vi "Create SG Power Meter Accessor.vi"(0 "SG Path":refnum<class "SG Abstract Path.lvclass">, 11 "error in":errorcluster) -> (4 "SG Path PM Accessor out":refnum<class "SG Path PM Accessor Base.lvclass">, 15 "error out":errorcluster)   [LabVIEW 2023, in "RFFixtureCharact.Instruments.lvlib" / "Power Meter Factory.lvclass"]
uses:
  Power Meter Factory.lvclass
  SG Path PM Accessor Base/SG Path PM Accessor Base.lvclass
  Public/Base Classes/Scalar/SG Abstract Path/SG Abstract Path.lvclass
  SG Path Simulated PM Accessor/SG Path Simulated PM Accessor.lvclass
  C:/srd-semi-rfcal-software/AuxTools/STSRFFixtureCharactUtility/Source/Code Modules/Fixture/Instruments/Power Meter/SG Path PM Accessor Base/SG Path PM Accessor Base.lvclass
  Simulated/Simulated Power Meter.lvclass
  C:/srd-semi-rfcal-software/AuxTools/STSRFFixtureCharactUtility/Source/Code Modules/Fixture/Instruments/Power Meter/Power Meter Base/Power Meter Base.lvclass
  13e43a11-3f49-451d-9662-7e96f715d9cd.vi
  <vilib>/Utility/error.llb/Trim Whitespace One-Sided.vi
  Common/Data Cache/Settings Dictionary/Setting Keys.vi
  <vilib>/Comparison/Equal/Equal Functor/Equal Functor.lvclass
  Power Meter Base/Power Meter Base.lvclass
  Power Meter Factory.lvclass/Power Meter Factory.ctl
  Common/RFCalAndFixtureCharact.Common.lvlib
  C:/srd-semi-rfcal-software/AuxTools/STSRFFixtureCharactUtility/Source/Code Modules/Fixture/Instruments/Power Meter/SG Path Simulated PM Accessor/SG Path Simulated PM Accessor.lvclass
  C:/srd-semi-rfcal-software/AuxTools/STSRFFixtureCharactUtility/Source/Code Modules/Fixture/Instruments/Power Meter/Simulated/Simulated Power Meter.lvclass
  C:/srd-semi-rfcal-software/AuxTools/STSRFFixtureCharactUtility/Source/Code Modules/Fixture/Public/Base Classes/Scalar/Scalar Path/Scalar Path.lvclass
  C:/srd-semi-rfcal-software/AuxTools/STSRFFixtureCharactUtility/Source/Code Modules/Common/Base Classes/Path/Path.lvclass
  C:/srd-semi-rfcal-software/AuxTools/STSRFFixtureCharactUtility/Source/Code Modules/Fixture/Public/Base Classes/Scalar/SG Abstract Path/SG Abstract Path.lvclass
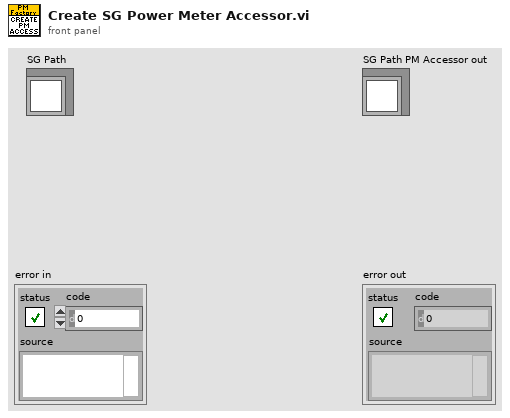
[diagram p1: front panel]
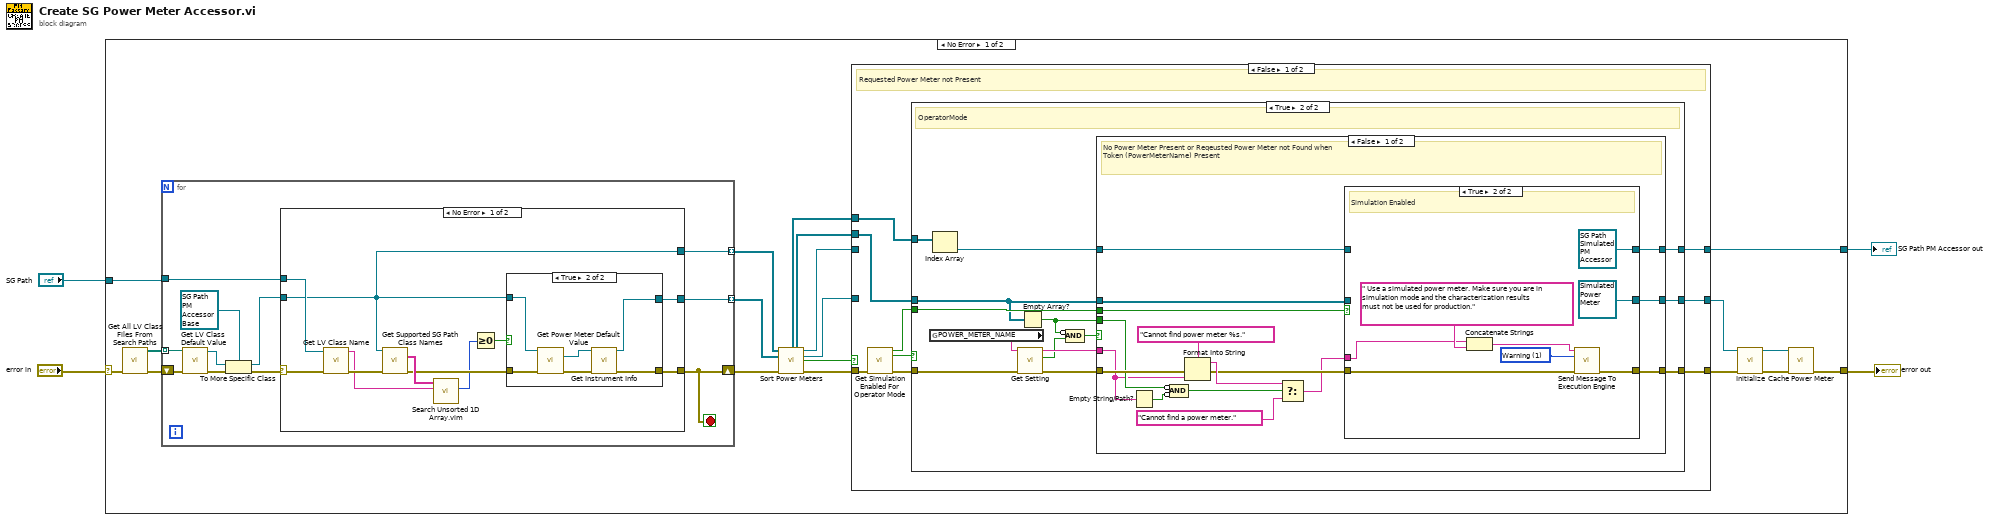
[diagram p0: block diagram]
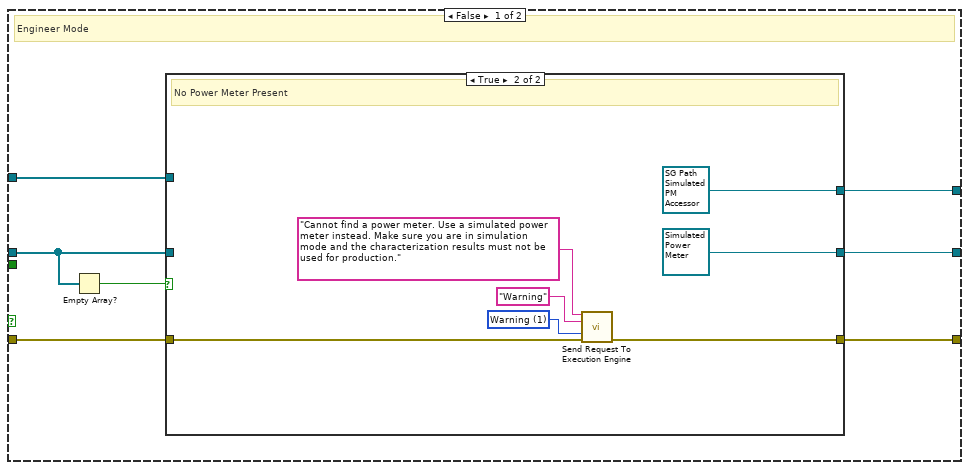
[diagram p2: hidden frame]
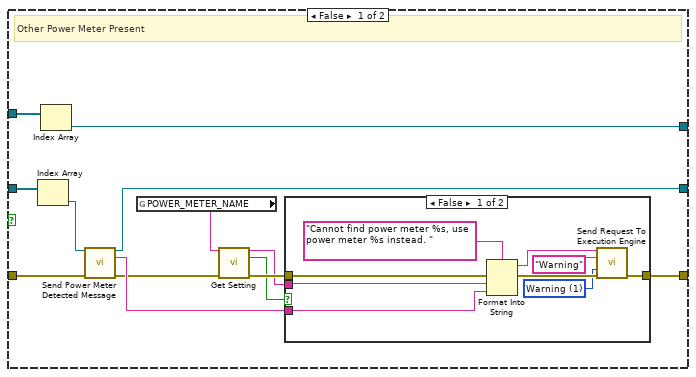
[diagram p3: hidden frame]
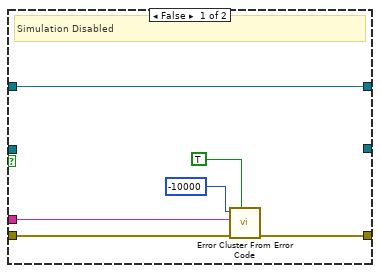
[diagram p5: hidden frame]
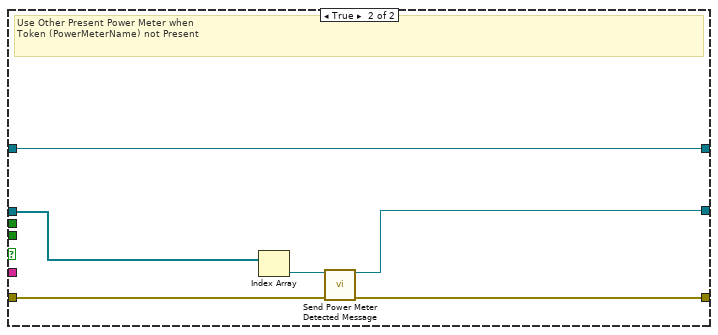
[diagram p6: hidden frame]
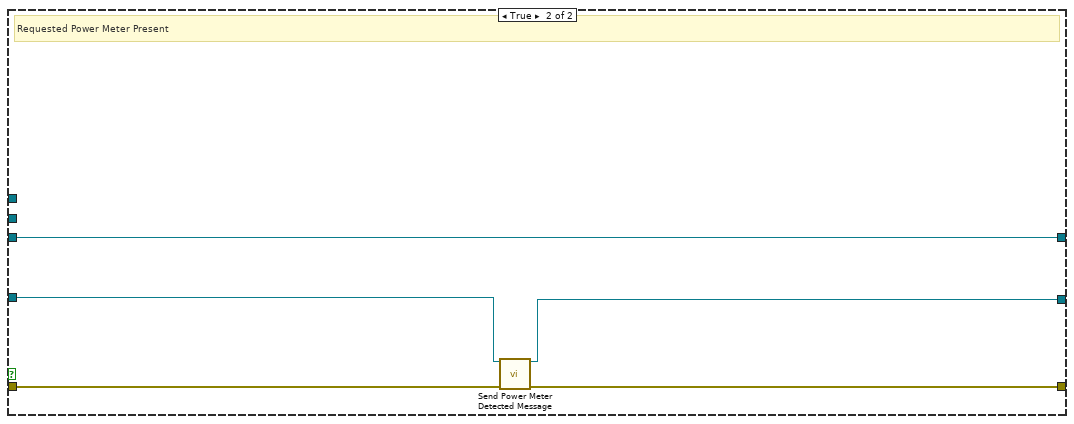
[diagram p7: hidden frame]
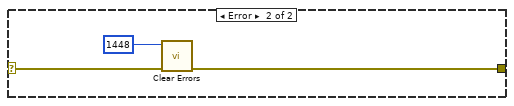
[diagram p9: hidden frame]
diagram:
  n1 = case shown="No Error" "error in" {
    selector: "error in" -> [w23 w157]
    tunnel: [w5 w157] -> w3
    tunnel: "SG Path" -> [w20 _]
    tunnel: [w19 _] -> w1
    frame No Error {
      n2 = call "Get All LV Class Files From Search Paths.vi"("error in (no error)"=w23) -> ("All Files in Dir"=w21:path[], "error out"=w22:errorcluster)  [unwired: 13 in]
      n3 = for {
        shift-right: [w128] -> w14
        shift-left: w22 -> [w135]
        tunnel: w21 -> [w133] mode=indexing
        tunnel: [w126] -> w17 mode=indexing
        tunnel: w20 -> [w129]
        tunnel: [w125] -> w18 mode=indexing
        stop <- w128 stop-if-true
        n4 = call <vilib>:"Get LV Class Default Value.vi"("error in (no error)"=w135, "class path"=w133) -> ("error out"=w134:errorcluster, "object"=w132:refnum<class>)  [unwired: 8 in]
        n5 = To More Specific Class(target class=refnum<class "SG Path PM Accessor Base.lvclass"> refnum ("RFFixtureCharact.Instruments.lvlib:SG Path PM Accessor Base.lvclass"), reference=w132, error in=w134) -> (specific class reference=w131:refnum<class "SG Path PM Accessor Base.lvclass">, error out=w130:errorcluster)
        n6 = case shown="No Error" w130 {
          selector: w130 -> [w146 w155]
          tunnel: [w142 w154] -> w128
          tunnel: w131 -> [w136 _]
          tunnel: [w143 _] -> w126
          tunnel: w129 -> [w145 _]
          tunnel: [w136 _] -> w125
          frame No Error {
            n7 = call <vilib>:"Get LV Class Name.vi"("error in (no error)"=w146, "object"=w145) -> ("error out"=w144:errorcluster, "class name"=w140:string)  [unwired: 8 in]
            n8 = call-dynamic "Get Supported SG Path Class Names.vi"("SG Path PM Accessor in"=w136, "error in"=w144) -> ("Supported SG Path Class Names"=w141:string[], "error out"=w139:errorcluster)  [unwired: 11 in, 1 out]
            n9 = call "Search Unsorted 1D Array.vim"("element"=w140, "unsorted 1D array"=w141) -> ("index of element"=w138:i32)  [unwired: 9 in]
            n10 = Greater Or Equal To 0?(x=w138) -> (x >= 0?=w137:bool)
            n11 = case shown="True" w137 {
              tunnel: w136 -> [_ w153]
              tunnel: [_ w151] -> w143
              tunnel: w139 -> [w147 w150]
              tunnel: [w147 w148] -> w142
              frame False {
              }
              frame True {
                n12 = call-dynamic "Get Power Meter Default Value.vi"("SG Path PM Accessor in"=w153, "error in (no error)"=w150) -> ("Power Meter out"=w149:refnum<class "Power Meter Base.lvclass">, "error out"=w152:errorcluster)  [unwired: 11 in, 1 out]
                n13 = call-dynamic "Get Instrument Info.vi"("Power Meter Base in"=w149, "error in (no error)"=w152) -> ("Power Meter Base out"=w151:refnum<class "Power Meter Base.lvclass">, "error out"=w148:errorcluster)  [unwired: 12 in]
              }
            }
          }
          frame Error {
            n14 = call <vilib>:"Clear Errors.vi"("error in (no error)"=w155, "specific error code to clear (0: all)"=1448) -> ("error out"=w154:errorcluster)  [unwired: 4 in, 1 out]
          }
        }
      }
      n15 = call "Sort Power Meters.vi"("SG Path PM Accessor Base Array in"=w18, "Power Meter Base Array in"=w17, "error in"=w14) -> ("All Present SG Path PMs Except Requested"=w13:refnum<class "SG Path PM Accessor Base.lvclass">[], "All Present PMs Except Requested"=w12:refnum<class "Power Meter Base.lvclass">[], "Requested SG Path PM Accessor"=w16:refnum<class "SG Path PM Accessor Base.lvclass">, "Requested PM"=w15:refnum<class "Power Meter Base.lvclass">, "Requested PM Found?"=w10:bool, "error out"=w11:errorcluster)  [unwired: 7 in]
      n16 = case shown="False" w10 {
        tunnel: [w32 w124] -> w19
        tunnel: [w31 w122] -> w7
        tunnel: w16 -> [_ w124]
        tunnel: w11 -> [w30 w123]
        tunnel: w15 -> [_ w121]
        tunnel: w13 -> [w25 _]
        tunnel: w12 -> [w26 _]
        tunnel: [w24 w120] -> w9
        frame False {
          # "Requested Power Meter not Present"
          n17 = call "Get Simulation Enabled For Operator Mode.vi"("error in (no error)"=w30) -> ("Use Simulated Instrument?"=w29:bool, "Use Operator Mode?"=w28:bool, "error out"=w27:errorcluster)  [unwired: 12 in]
          n18 = case shown="True" w28 {
            tunnel: w29 -> [_ w83]
            tunnel: w27 -> [w39 w76]
            tunnel: [w38 w82] -> w32
            tunnel: [w34 w81] -> w31
            tunnel: w26 -> [w36 w74]
            tunnel: w25 -> [w35 w80]
            tunnel: [w33 w78] -> w24
            frame False {
              # "Engineer Mode"
              n19 = Empty Array?(array=w36) -> (empty?=w37:bool)
              n20 = case shown="True" w37 {
                tunnel: w39 -> [w45 w66]
                tunnel: [w40 w69] -> w34
                tunnel: [w51 refnum<class "SG Path Simulated PM Accessor.lvclass"> refnum ("RFFixtureCharact.Instruments.lvlib:SG Path Simulated PM Accessor.lvclass")] -> w38
                tunnel: w36 -> [w44 _]
                tunnel: w35 -> [w52 _]
                tunnel: [w50 refnum<class "Simulated Power Meter.lvclass"> refnum ("PM Simulated in")] -> w33
                frame False {
                  # "Other Power Meter Present"
                  n21 = Index Array(array=w44) -> (element=w43:refnum<class "Power Meter Base.lvclass">)  [unwired: 1 in]
                  n22 = Index Array(array=w52) -> (element=w51:refnum<class "SG Path PM Accessor Base.lvclass">)  [unwired: 1 in]
                  n23 = call "Send Power Meter Detected Message.vi"("Power Meter in"=w43, "error in"=w45) -> ("Power Meter out"=w50:refnum<class "Power Meter Base.lvclass">, "Active Instrument Info String"=w42:string, "error out"=w41:errorcluster)  [unwired: 11 in]
                  n24 = global read "Setting Keys.vi" "POWER_METER_NAME"() -> (w49:string)
                  n25 = call "Get Setting.vi"("Setting name"=w49, "error in (no error)"=w41) -> ("Setting value out"=w46:string, "Setting empty or not found?"=w47:bool, "error out"=w48:errorcluster)  [unwired: 11 in]
                  n26 = case shown="False" w47 {
                    tunnel: w48 -> [w60 w62]
                    tunnel: w42 -> [w53 _]
                    tunnel: [w55 w62] -> w40
                    tunnel: w46 -> [w54 _]
                    frame False {
                      w56 = 1 items=["Info", "Warning", "Error", "Action"] ("Request Content Type")
                      n27 = Format Into String(format string="Cannot find power meter %s, use power meter %s instead. " ("message"), error in=w60, w54, w53) -> (resulting string=w58:string, error out=w57:errorcluster)  [unwired: 1 in]
                      n28 = call "Send Request To Execution Engine.vi"("Request Message"=w58, "Request Header"="Warning", "Request Content Type"=w56, "error in (no error)"=w57) -> ("error out"=w55:errorcluster)  [unwired: 10 in, 1 out]
                    }
                    frame True {
                    }
                  }
                }
                frame True {
                  w67 = 1 items=["Info", "Warning", "Error", "Action"] ("RequestContentType")
                  # "No Power Meter Present"
                  n29 = call "Send Request To Execution Engine.vi"("Request Message"="Cannot find a power meter. Use a simulated power meter instead. Make sure you are in simulation mode and the characterization results must not be used for production." ("message"), "Request Header"="Warning" ("headerText"), "Request Content Type"=w67, "error in (no error)"=w66) -> ("error out"=w69:errorcluster)  [unwired: 10 in, 1 out]
                }
              }
            }
            frame True {
              # "OperatorMode"
              n30 = global read "Setting Keys.vi" "POWER_METER_NAME"() -> (w77:string)
              n31 = Index Array(array=w80) -> (element=w79:refnum<class "SG Path PM Accessor Base.lvclass">)  [unwired: 1 in]
              n32 = call "Get Setting.vi"("Setting name"=w77, "error in (no error)"=w76) -> ("Setting value out"=w72:string, "Setting empty or not found?"=w71:bool, "error out"=w75:errorcluster)  [unwired: 11 in]
              n33 = Empty Array?(array=w74) -> (empty?=w70:bool)
              n34 = Compound Arithmetic op=AND(invert w70, w71) -> (w73:bool)
              n35 = case shown="False" w73 {
                tunnel: w83 -> [w99 _]
                tunnel: [w98 w115] -> w82
                tunnel: [w97 w114] -> w81
                tunnel: w79 -> [w96 w115]
                tunnel: [w95 w117] -> w78
                tunnel: w75 -> [w88 w118]
                tunnel: w74 -> [w94 w116]
                tunnel: w72 -> [w85 _]
                tunnel: w70 -> [w86 _]
                frame False {
                  # "No Power Meter Present or Reqeusted Power Meter not Found when \nToken (PowerMeterName) Present"
                  n36 = Empty String/Path?(string/path=w85) -> (empty?=w92:bool)
                  n37 = Compound Arithmetic op=AND(invert w86, invert w92) -> (w91:bool)
                  n38 = Format Into String(format string="Cannot find power meter %s." ("message"), error in=w88, w85) -> (resulting string=w90:string, error out=w87:errorcluster)  [unwired: 1 in]
                  n39 = Select(t=w90, s=w91, f="Cannot find a power meter." ("message")) -> (s? t:f=w84:string)
                  n40 = case shown="True" w99 {
                    tunnel: [w105 refnum<class "SG Path Simulated PM Accessor.lvclass"> refnum ("RFFixtureCharact.Instruments.lvlib:SG Path Simulated PM Accessor.lvclass")] -> w98
                    tunnel: w87 -> [w101 w107]
                    tunnel: [w104 w113] -> w97
                    tunnel: w96 -> [w105 _]
                    tunnel: w94 -> [_ _]
                    tunnel: [_ refnum<class "Simulated Power Meter.lvclass"> refnum ("PM Simulated in")] -> w95
                    tunnel: w84 -> [w100 w106]
                    frame False {
                      # "Simulation Disabled"
                      n41 = call <vilib>:"Error Cluster From Error Code.vi"("show call chain? (False)"=TRUE, "error in (no error)"=w101, "error message (\"\")"=w100, "error code (0)"=-10000) -> ("error out"=w104:errorcluster)  [unwired: 5 in]
                    }
                    frame True {
                      w112 = 1 items=["Info", "Warning", "Error", "Action"] ("RequestContentType")
                      # "Simulation Enabled"
                      n42 = Concatenate Strings(w106, " Use a simulated power meter. Make sure you are in simulation mode and the characterization results must not be used for production." ("message")) -> (w108:string)
                      n43 = call "Send Message To Execution Engine.vi"("Message"=w108, "Message Type"=w112, "error in (no error)"=w107) -> ("error out"=w113:errorcluster)  [unwired: 12 in]
                    }
                  }
                }
                frame True {
                  # "Use Other Present Power Meter when \nToken (PowerMeterName) not Present"
                  n44 = Index Array(array=w116) -> (element=w119:refnum<class "Power Meter Base.lvclass">)  [unwired: 1 in]
                  n45 = call "Send Power Meter Detected Message.vi"("Power Meter in"=w119, "error in"=w118) -> ("Power Meter out"=w117:refnum<class "Power Meter Base.lvclass">, "error out"=w114:errorcluster)  [unwired: 11 in, 1 out]
                }
              }
            }
          }
        }
        frame True {
          # "Requested Power Meter Present"
          n46 = call "Send Power Meter Detected Message.vi"("Power Meter in"=w121, "error in"=w123) -> ("Power Meter out"=w120:refnum<class "Power Meter Base.lvclass">, "error out"=w122:errorcluster)  [unwired: 11 in, 1 out]
        }
      }
      n47 = call-dynamic "Initialize.vi"("Power Meter Base in"=w9, "error in (no error)"=w7) -> ("Power Meter Base out"=w8:refnum<class "Power Meter Base.lvclass">, "error out"=w6:errorcluster)  [unwired: 12 in]
      n48 = call "Cache Power Meter.vi"("Power Meter Base in"=w8, "error in (no error)"=w6) -> ("error out"=w5:errorcluster)  [unwired: 12 in, 1 out]
    }
    frame Error {
    }
  }
  "SG Path PM Accessor out" <- w1
  "error out" <- w3
